vi "update.Defer.vi"(5 "Defer Panel Updates":bool, 7 "bus in":T1, 8 "error in":errorcluster) -> (0 "error out":errorcluster)   [LabVIEW 2020]
uses:
  bus.ctl
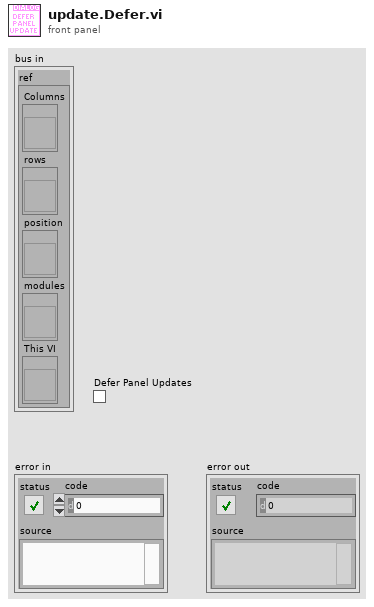
[diagram p1: front panel]
types:
  T1 = typedef "bus.ctl" = cluster{"ref":cluster{"Columns":refnum<vi>, "rows":refnum<vi>, "position":refnum<vi>, "modules":refnum<vi>, "This VI":refnum<vi>}}
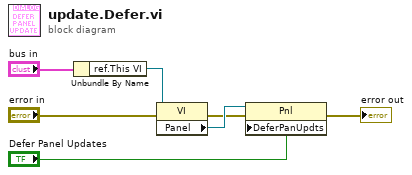
[diagram p0: block diagram]
diagram:
  n1 = Unbundle By Name("bus in") -> ("ref.This VI"=w1:refnum<vi>)
  n2 = property class="VI"(reference=w1, error in="error in") -> (error out=w3:errorcluster, "Panel"=w6:refnum<vi>)  [unwired: 1 out]
  n3 = property class="Pnl"(reference=w6, error in=w3, "DeferPanUpdts"="Defer Panel Updates") -> (error out=→"error out":errorcluster)  [unwired: 1 out]
